vi "GetComPortList.vi"(8 "In":errorcluster) -> (0 "Out":errorcluster, 2 "COM_List":string[](array[string]))   [LabVIEW 2019]
uses:
  <vilib>/Instr/_visa.llb/VISA Find Search Mode.ctl
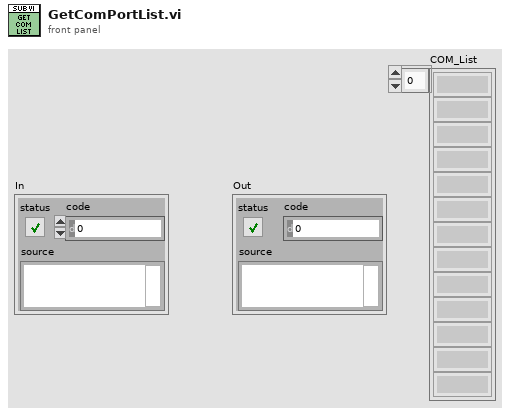
[diagram p1: front panel]
types:
  T1 = typedef "VISA Find Search Mode.ctl" = u32
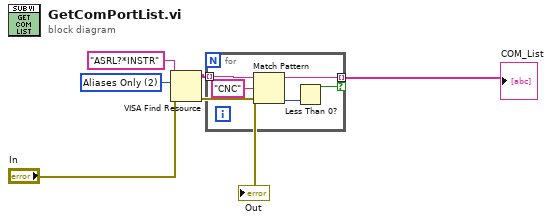
[diagram p0: block diagram]
diagram:
  w6 = T1 2 items=["Canonical Names Only"=0, "Aliases Only"=2, "Include Matching Aliases"=3, "Include All Aliases"=4] ("Search Mode")
  n1 = VISA Find Resource(8:"In", 10:w6, 11:"ASRL?*INSTR" ("expression (\"?*\")")) -> (0:→"Out":errorcluster, 3:w4:string[])  [unwired: 1 out]
  n2 = for {
    tunnel: w4 -> [w9] mode=indexing
    tunnel: [w9] -> w3 mode=indexing if=w7
    n3 = Match Pattern(string=w9, regular expression="CNC") -> (offset past match=w8:i32)  [unwired: 1 in, 3 out]
    n4 = Less Than 0?(x=w8) -> (x < 0?=w7:bool)
  }
  "COM_List" <- w3
